vi "Mutex Get Priority Ceiling.vi"(8 "error in (no error)":errorcluster, 11 "Mutex in":T1) -> (0 "error out":errorcluster, 2 "priority ceiling":i32, 3 "Mutex out":T1)   [LabVIEW 2013, in "Linux RT IPC.lvlib" / "POSIX Threads.lvlib" / "Mutex.lvclass"]
doc: "Calls pthread_mutex_getprioceiling() on the pthread mutex object encapsulated by Mutex.\n\nThis VI returns the current priority ceiling for the provided mutex. The priority ceiling refers to the maximum priority that the mutex can be elevated to in the event of a priority inversion.\n\nRefer to online POSIX documentation for more information."
uses:
  Mutex.lvclass
  Controls/reference.ctl
  POSIX Thread Object/POSIX Thread Object.lvclass/POSIX Thread Object.ctl
  POSIX Thread Object/Private VIs/libpthread path.vi
  POSIX Thread Object/Private VIs/get pthread error.vi
  POSIX Thread Object/POSIX Thread Object.lvclass
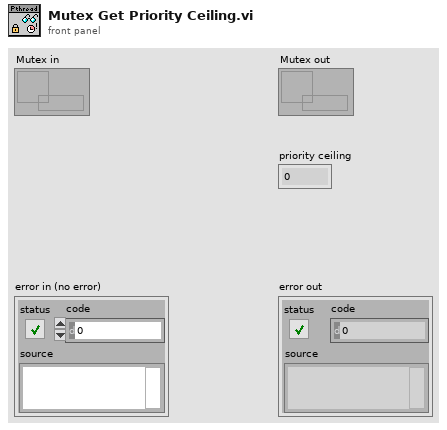
[diagram p1: front panel]
types:
  T1 = typedef "Linux RT IPC.lvlib/POSIX Threads.lvlib/Mutex.lvclass/reference.ctl" = refnum<data-value>
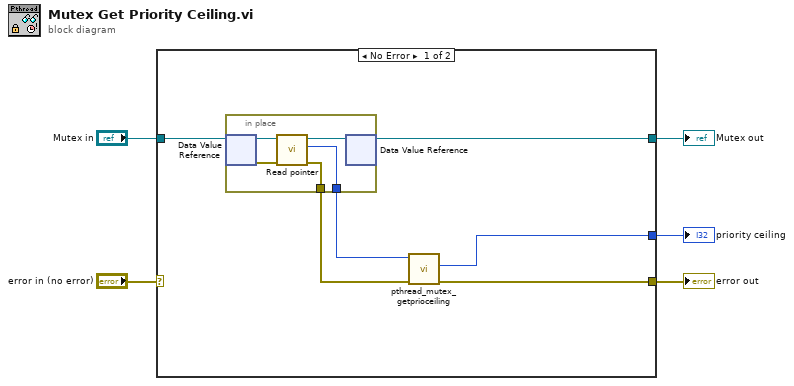
[diagram p0: block diagram]
diagram:
  n1 = case shown="No Error" "error in (no error)" {
    selector: "error in (no error)" -> [_ w18]
    tunnel: [w9 w18] -> w4
    tunnel: "Mutex in" -> [w11 w17]
    tunnel: [w10 w17] -> w2
    tunnel: [w6 _] -> w1
    frame No Error {
      n2 = in-place {
        in-place-border: [w13] -> w8
        in-place-border: [w12] -> w7
        n3 = in-place-dvr #1(w11) -> (w16:refnum<class "Mutex.lvclass">, w14:errorcluster)
        n4 = call "Read pointer.vi"("error in (no error)"=w14, "POSIX Thread Object in"=w16) -> ("error out"=w13:errorcluster, "pointer"=w12:u64, "POSIX Thread Object out"=w15:refnum<class "Mutex.lvclass">)  [unwired: 7 in]
        n5 = in-place-dvr #1(w15) -> (w10:T1)  [unwired: 1 out]
      }
      n6 = call "pthread_mutex_getprioceiling.vi"("error in (no error)"=w8, "mutex ptr in"=w7) -> ("error out"=w9:errorcluster, "priority ceiling"=w6:i32)  [unwired: 7 in, 1 out]
    }
    frame Error {
    }
  }
  "Mutex out" <- w2
  "error out" <- w4
  "priority ceiling" <- w1
